vi "RemoveFrontEnd.vi"(8 "error in (no error)":errorcluster, 11 "FE Name":string="RemoveFrontEnd") -> (0 "error out":errorcluster, 3 "TestSetDef":T1={"General"={"ID"=0, "Model"="", "Dual Port?"=FALSE, "Options"="", "Options"={"E"=FALSE, "K"=FALSE, "H"=FALSE, "W"=FALSE, "F"=FALSE}, "Cal File"=path ""}, "Receiver"={"Fstart, MHz"=0.0, "Fstop MHz"=0.0, "Fstep MHz"=0.0, "IF, MHz"=0.0}, "RX Band"={"Fstart, MHz"=0.0, "Fstop MHz"=0.0}, "TX 1"={"Fstart, MHz"=0.0, "Fstop MHz"=0.0, "Pmax, dBm"=0.0, "Pstep, dB"=0.0}, "TX 2"={"Fstart, MHz"=0.0, "Fstop MHz"=0.0, "Pmax, dBm"=0.0, "Pstep, dB"=0.0}, "Low-side?"=TRUE})   [LabVIEW 2011]
uses:
  Test Set Definition.ctl
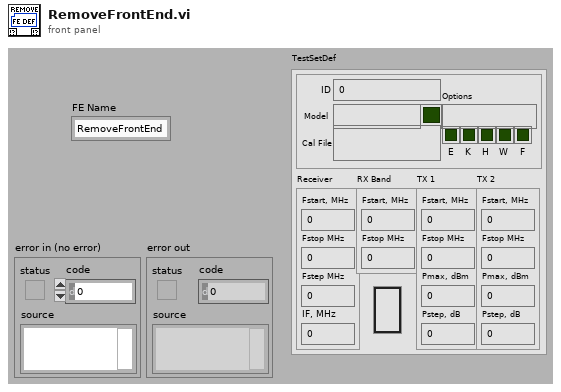
[diagram p1: front panel]
types:
  T1 = typedef "Test Set Definition.ctl" = cluster{"General":cluster{"ID":u32, "Model":string, "Dual Port?":bool, "Options":string, "Options":cluster{"E":bool, "K":bool, "H":bool, "W":bool, "F":bool}, "Cal File":path}, "Receiver":cluster{"Fstart, MHz":dbl, "Fstop MHz":dbl, "Fstep MHz":dbl, "IF, MHz":dbl}, "RX Band":cluster{"Fstart, MHz":dbl, "Fstop MHz":dbl}, "TX 1":cluster{"Fstart, MHz":dbl, "Fstop MHz":dbl, "Pmax, dBm":dbl, "Pstep, dB":dbl}, "TX 2":cluster{"Fstart, MHz":dbl, "Fstop MHz":dbl, "Pmax, dBm":dbl, "Pstep, dB":dbl}, "Low-side?":bool}
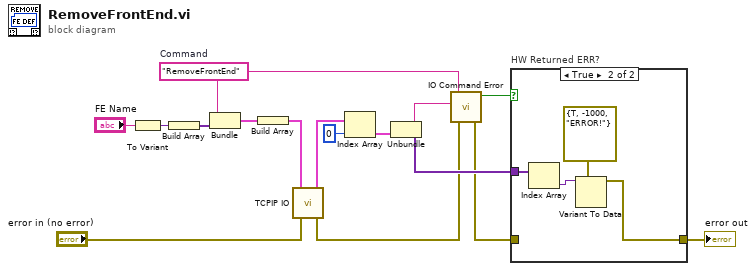
[diagram p0: block diagram]
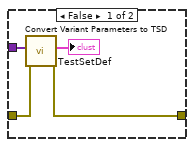
[diagram p2: hidden frame]
diagram:
  w13 = "RemoveFrontEnd"  # Command
  n1 = To Variant(anything="FE Name") -> (Variant=w2:variant)
  n2 = Build Array(w2) -> (w1:variant[])
  n3 = Bundle("Command"=w13, w1) -> (w15:cluster{"Command":string, variant[]})  [unwired: 1 out]
  n4 = Build Array(w15) -> (w12:cluster{"Command":string, variant[]}[])
  n5 = call "TCPIP IO.vi"("error in (no error)"="error in (no error)", "Commands"=w12) -> ("error out"=w6:errorcluster, "Responses"=w11:cluster{string, variant[]}[])  [unwired: 1 in, 3 out]
  n6 = Index Array(array=w11, index=0) -> (element=w10:cluster{string, variant[]})
  n7 = Unbundle(w10) -> (w9:string, w8:variant[])
  n8 = call "IO Command Error.vi"("error in (no error)"=w6, "Command Returned (\"\")"=w9, "Command Sent (\"\")"=w13) -> ("error out"=w5:errorcluster, "HW ERR?"=w7:bool)  [unwired: 3 out]
  n9 = case "HW Returned ERR?" shown="True" w7 {
    tunnel: w5 -> [w20 _]
    tunnel: w8 -> [w17 w22]
    tunnel: [w19 w21] -> w4
    frame False {
      n10 = call "Convert Variant Parameters to TSD.vi"("error in"=w20, "Variant Parameter Array"=w17) -> ("error out"=w19:errorcluster, "TestSetDef"=→"TestSetDef":T1)  [unwired: 8 out]
    }
    frame True {
      n11 = Index Array(array=w22) -> (element=w24:variant)  [unwired: 1 in]
      n12 = Variant To Data(type=errorcluster {"status"=TRUE, "code"=-1000, "source"="ERROR!"} ("error out"), Variant=w24) -> (data=w21:errorcluster)  [unwired: 1 in, 1 out]
    }
  }
  "error out" <- w4
